vi "Turn.vi"(8 "Acceptable Error (Degrees)":dbl=1.0, 10 "Heading Change (Degrees)":dbl) -> (0 "Actual Heading (Degrees)":dbl(knob)=0.4937889940289276 scale=-180.0..180.0, 3 "Motor DevRef":T1={"DeviceStatus"={"status"=FALSE, "code"=0, "source"=""}, "Type"=enum."PWM", "PWM"={"Digital Module"=enum."Digital Module 1", "PWM Channel"=enum."Invalid", "DeadBand"={"Name"="", "maxPositivePwm"=0, "minPositivePwm"=0, "centerPwm"=0, "maxNegativePwm"=0, "minNegativePwm"=0, "angularRange"=0}}, "CAN"={"Device Number"=0, "Control Mode"=enum."Percent VBus", "Semaphore"=refnum, "Max Vout"=12.0}, "Invert"=FALSE, "TransformRef"=refnum, "InvTransformRef"=refnum})   [LabVIEW 2012]
uses:
  <vilib>/Rock Robotics/WPI/MotorControl/WPI_MotorControlDeviceRef.ctl
  <vilib>/Rock Robotics/SystemInterfaces/Typedef/FPGA_TypedefDigitalModule.ctl
  <vilib>/Rock Robotics/SystemInterfaces/DIO/FPGA_DIOPWMChannel.ctl
  <vilib>/Rock Robotics/WPI/PWM/WPI_PWMDeadband.ctl
  <vilib>/Rock Robotics/WPI/CAN/Jaguar/SubVIs/WPI_CANJaguar_ControlMode.ctl
  <vilib>/Rock Robotics/WPI/PWM/WPI_PWMTransform_ConPane.ctl
  Robot Global Data.vi
panel:
  in  "Rotation Speed":dbl=0.3
  out "Rotation":dbl
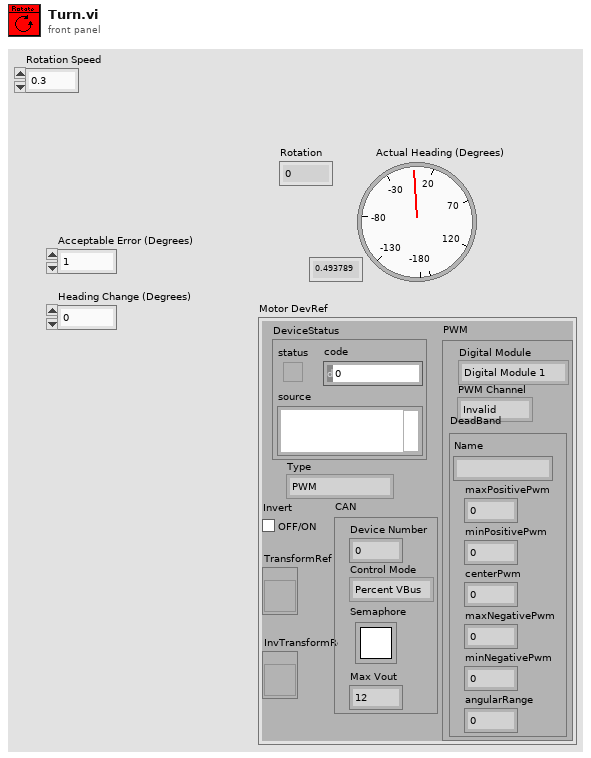
[diagram p1: front panel]
types:
  T1 = typedef "WPI_MotorControlDeviceRef.ctl" = cluster{"DeviceStatus":errorcluster, "Type":enum16{"PWM", "CAN"}, "PWM":cluster{"Digital Module":T2, "PWM Channel":T3, "DeadBand":T4}, "CAN":cluster{"Device Number":u8, "Control Mode":T5, "Semaphore":T6, "Max Vout":dbl}, "Invert":bool, "TransformRef":T7, "InvTransformRef":T7}
  T2 = typedef "FPGA_TypedefDigitalModule.ctl" = enum16{"Digital Module 1", "Digital Module 2"}
  T3 = typedef "FPGA_DIOPWMChannel.ctl" = enum8{"PWM 1", "PWM 2", "PWM 3", "PWM 4", "PWM 5", "PWM 6", "PWM 7", "PWM 8", "PWM 9", "PWM 10", "Invalid"}
  T4 = typedef "WPI_PWMDeadband.ctl" = cluster{"Name":string, "maxPositivePwm":i32, "minPositivePwm":i32, "centerPwm":i32, "maxNegativePwm":i32, "minNegativePwm":i32, "angularRange":u16}
  T5 = typedef "WPI_CANJaguar_ControlMode.ctl" = enum8{"Percent VBus", "Current", "Speed", "Position", "Voltage"}
  T6 = typedef "Semaphore RefNum" = refnum<k1>
  T7 = typedef "WPI_PWMTransform_ConPane.ctl" = refnum<vi>
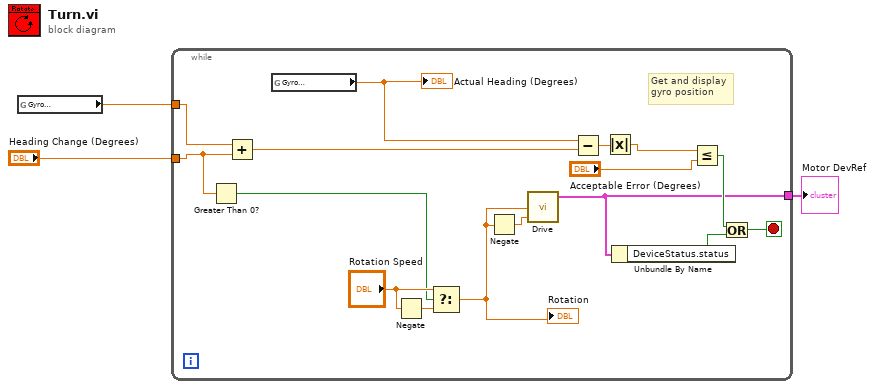
[diagram p0: block diagram]
diagram:
  n1 = global read "Robot Global Data.vi" "Gyro\nAngle"() -> (w2:dbl)
  n2 = while {
    tunnel: "Heading Change (Degrees)" -> [w5]
    tunnel: [w9] -> w1
    tunnel: w2 -> [w13]
    stop <- w19 stop-if-true
    # "Get and display\ngyro position"
    n3 = Greater Than 0?(x=w5) -> (x > 0?=w4:bool)
    n4 = Add(x=w13, y=w5) -> (x+y=w11:dbl)
    n5 = global read "Robot Global Data.vi" "Gyro\nAngle"() -> (w10:dbl)
    "Actual Heading (Degrees)" <- w10
    n6 = Negate(x="Rotation Speed") -> (-x=w8:dbl)
    n7 = Select(t="Rotation Speed", s=w4, f=w8) -> (s? t:f=w6:dbl)
    "Rotation" <- w6
    n8 = Negate(x=w6) -> (-x=w12:dbl)
    n9 = call "Drive.vi"("Right Motor IN"=w12, "Left Motor IN"=w6) -> ("Motor DevRef"=w9:T1)  [unwired: 3 in]
    n10 = Subtract(x=w10, y=w11) -> (x-y=w18:dbl)
    n11 = Absolute Value(x=w18) -> (abs(x)=w17:dbl)
    n12 = Unbundle By Name(w9) -> ("DeviceStatus.status"=w15:bool)
    n13 = Less Or Equal?(x=w17, y="Acceptable Error (Degrees)") -> (x <= y?=w14:bool)
    n14 = Or(x=w14, y=w15) -> (x .or. y?=w19:bool)
  }
  "Motor DevRef" <- w1
